vi "Calculator.vi"() -> ()   [LabVIEW 2019]
panel:
  in  "Stop Button":bool
  out "Display":string
  in  "Cluster":T1
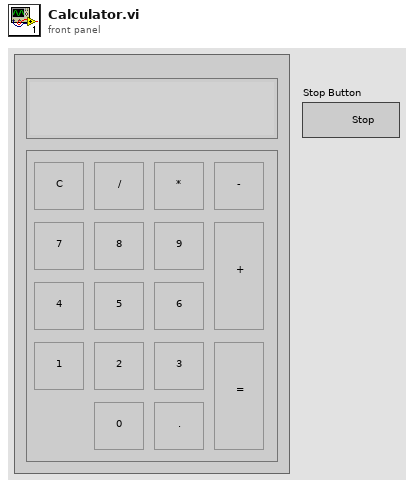
[diagram p1: front panel]
types:
  T1 = cluster{"Equal":bool, "Add":bool, "Decimal":bool, "Zero":bool, "Three":bool, "Two":bool, "One":bool, "Six":bool, "Five":bool, "Four":bool, "Nine":bool, "Eight":bool, "Seven":bool, "Sub":bool, "Mul":bool, "Div":bool, "Clear":bool}
  T2 = enum16{"Sum", "Mul", "Div", "Sub", "Sin function"}
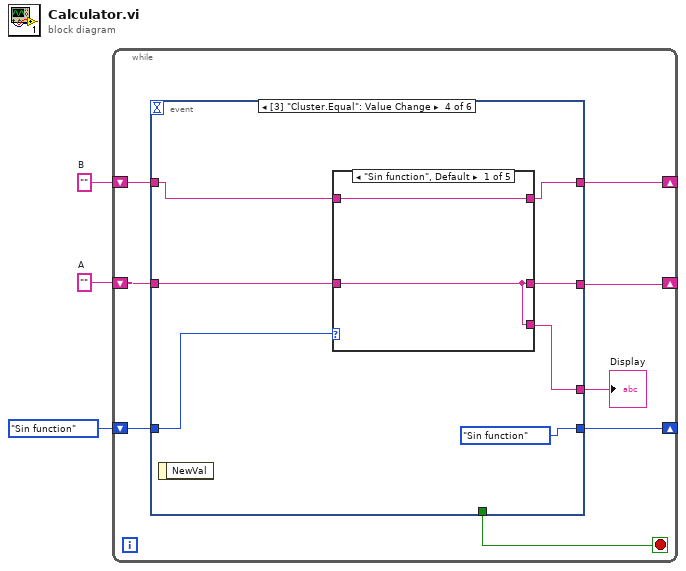
[diagram p0: block diagram]
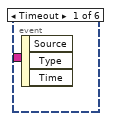
[diagram p2: hidden frame]
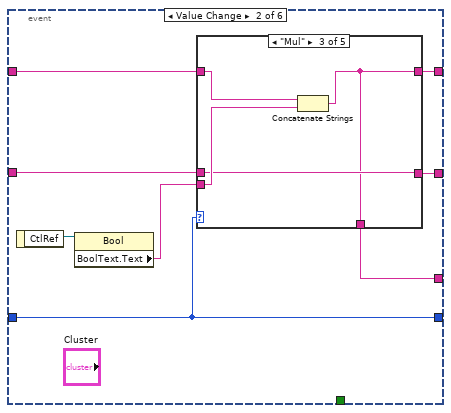
[diagram p3: hidden frame]
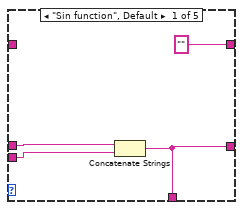
[diagram p4: hidden frame]
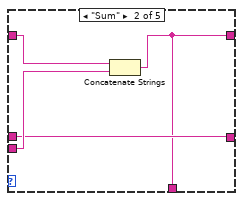
[diagram p5: hidden frame]
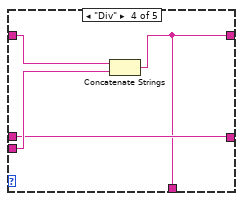
[diagram p6: hidden frame]
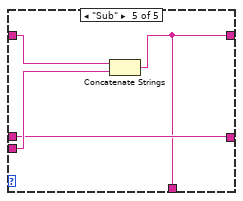
[diagram p7: hidden frame]
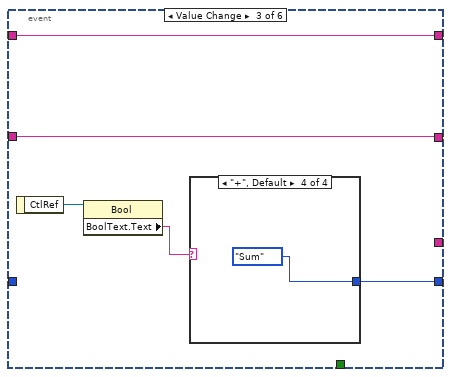
[diagram p8: hidden frame]
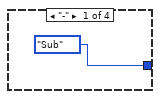
[diagram p9: hidden frame]
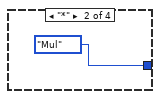
[diagram p10: hidden frame]
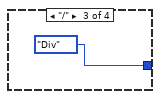
[diagram p11: hidden frame]
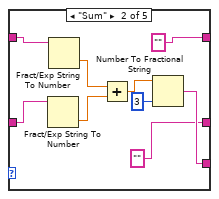
[diagram p12: hidden frame]
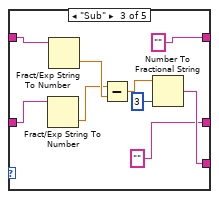
[diagram p13: hidden frame]
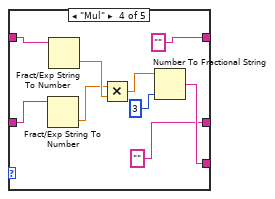
[diagram p14: hidden frame]
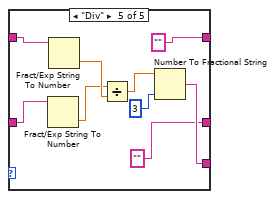
[diagram p15: hidden frame]
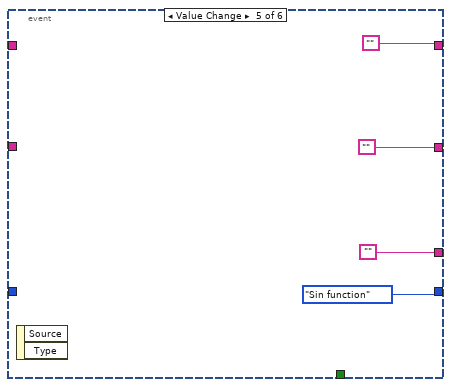
[diagram p16: hidden frame]
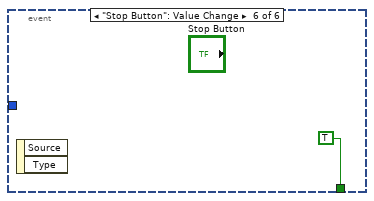
[diagram p17: hidden frame]
diagram:
  w2 = ""  # A
  w3 = ""  # B
  n1 = while {
    shift-right: [w5] -> _
    shift-left: w3 -> [w6]
    shift-right: [w8] -> _
    shift-left: w2 -> [w9]
    shift-right: [w10] -> _
    shift-left: T2."Sin function" -> [w11]
    stop <- w4 stop-if-true
    n2 = event shown="[3] \"Cluster.Equal\": Value Change" {
      selector: _ -> [_ _ _ _ _ _]
      dyn-events: _ -> [_ _ _ _ _ _]
      timeout: _ -> [_ _ _ _ _ _]
      tunnel: w11 -> [_ w19 _ w55 _ _]
      tunnel: [_ w19 w42 T2."Sin function" T2."Sin function" _] -> w10
      tunnel: w9 -> [_ w17 w40 w53 _ _]
      tunnel: [_ w15 w40 w52 "" _] -> w8
      tunnel: [_ w14 _ w49 "" _] -> w7
      tunnel: w6 -> [_ w13 w41 w51 _ _]
      tunnel: [_ w12 w41 w50 "" _] -> w5
      tunnel: [_ _ _ _ _ TRUE] -> w4
      event Timeout {
        n3 = event-data() -> ()  [unwired: 1 in, 3 out]
      }
      event "Cluster.Zero", "Cluster.One", "Cluster.Two", "Cluster.Three", "Cluster.Four", "Cluster.Five", "Cluster.Six", "Cluster.Seven", "Cluster.Eight", "Cluster.Nine", "Cluster.Decimal": Value Change {
        n4 = event-data() -> ("CtlRef"=w18:refnum<vi>)  [unwired: 1 in]
        n5 = property class="Bool"(reference=w18) -> ("BoolText.Text"=w16:string)  [unwired: 1 in, 2 out]
        n6 = case shown="\"Mul\"" w19 {
          tunnel: w17 -> [w23 w25 w29 w33 w37]
          tunnel: w16 -> [w22 w26 w30 w34 w38]
          tunnel: [w21 w25 w29 w33 w37] -> w15
          tunnel: [w21 w24 w28 w32 w36] -> w14
          tunnel: w13 -> [_ w27 w31 w35 w39]
          tunnel: ["" w24 w28 w32 w36] -> w12
          frame "Sin function", Default {
            n7 = Concatenate Strings(w23, w22) -> (w21:string)
          }
          frame "Sum" {
            n8 = Concatenate Strings(w27, w26) -> (w24:string)
          }
          frame "Mul" {
            n9 = Concatenate Strings(w31, w30) -> (w28:string)
          }
          frame "Div" {
            n10 = Concatenate Strings(w35, w34) -> (w32:string)
          }
          frame "Sub" {
            n11 = Concatenate Strings(w39, w38) -> (w36:string)
          }
        }
      }
      event "Cluster.Add", "Cluster.Sub", "Cluster.Mul", "Cluster.Div": Value Change {
        n12 = event-data() -> ("CtlRef"=w44:refnum<vi>)  [unwired: 1 in]
        n13 = property class="Bool"(reference=w44) -> ("BoolText.Text"=w43:string)  [unwired: 1 in, 2 out]
        n14 = case shown="\"+\", Default" w43 {
          tunnel: [T2."Sub" T2."Mul" T2."Div" T2."Sum"] -> w42
          frame "-" {
          }
          frame "*" {
          }
          frame "/" {
          }
          frame "+", Default {
          }
        }
      }
      event "Cluster.Equal": Value Change {
        n15 = event-data() -> ()  [unwired: 1 in, 1 out]
        n16 = case shown="\"Sin function\", Default" w55 {
          tunnel: w53 -> [w56 w62 w73 w82 w91]
          tunnel: [w56 "" "" "" ""] -> w52
          tunnel: w51 -> [w57 w63 w74 w83 w92]
          tunnel: [w57 "" "" "" ""] -> w50
          tunnel: [w56 w61 w72 w81 w90] -> w49
          frame "Sin function", Default {
          }
          frame "Sum" {
            n17 = Fract/Exp String To Number(string=w62) -> (number=w64:dbl)  [unwired: 3 in, 1 out]
            n18 = Fract/Exp String To Number(string=w63) -> (number=w66:dbl)  [unwired: 3 in, 1 out]
            n19 = Add(x=w66, y=w64) -> (x+y=w58:dbl)
            n20 = Number To Fractional String(number=w58, precision (6)=i16 3) -> (F-format string=w61:string)  [unwired: 2 in]
          }
          frame "Sub" {
            n21 = Fract/Exp String To Number(string=w73) -> (number=w68:dbl)  [unwired: 3 in, 1 out]
            n22 = Fract/Exp String To Number(string=w74) -> (number=w69:dbl)  [unwired: 3 in, 1 out]
            n23 = Subtract(x=w68, y=w69) -> (x-y=w67:dbl)
            n24 = Number To Fractional String(number=w67, precision (6)=i16 3) -> (F-format string=w72:string)  [unwired: 2 in]
          }
          frame "Mul" {
            n25 = Fract/Exp String To Number(string=w82) -> (number=w77:dbl)  [unwired: 3 in, 1 out]
            n26 = Fract/Exp String To Number(string=w83) -> (number=w78:dbl)  [unwired: 3 in, 1 out]
            n27 = Multiply(x=w77, y=w78) -> (x*y=w76:dbl)
            n28 = Number To Fractional String(number=w76, precision (6)=i16 3) -> (F-format string=w81:string)  [unwired: 2 in]
          }
          frame "Div" {
            n29 = Fract/Exp String To Number(string=w91) -> (number=w86:dbl)  [unwired: 3 in, 1 out]
            n30 = Fract/Exp String To Number(string=w92) -> (number=w87:dbl)  [unwired: 3 in, 1 out]
            n31 = Divide(x=w86, y=w87) -> (x/y=w85:dbl)
            n32 = Number To Fractional String(number=w85, precision (6)=i16 3) -> (F-format string=w90:string)  [unwired: 2 in]
          }
        }
      }
      event "Cluster.Clear": Value Change {
        n33 = event-data() -> ()  [unwired: 1 in, 2 out]
      }
      event "Stop Button": Value Change {
        n34 = event-data() -> ()  [unwired: 1 in, 2 out]
      }
    }
    "Display" <- w7
  }
